vi "Fastlite5216_Example.vi"() -> ()   [LabVIEW 2020]
uses:
  <vilib>/Analysis/baseanly.llb/Mean (DBL).vi
  Fastlite5216_VIs/Fastlite5216-VIs.lvlib
  <vilib>/Analysis/NI_AALBase.lvlib
panel:
  in  "Correct Elec. Dark Current":bool
  in  "MeasConfigData":T1={"StartPixel"=0, "StopPixel"=2047, "Integration Time"=0.005, "Integration Delay"=0.0, "Trigger Mode"=enum."Software", "N StoreToRam"=0} {"Integration Delay" min=-0.02; "StopPixel" max=4095 step=1; "StartPixel" max=4095 step=1}
  out "Spectrum":cluster{dbl[], "Spectral DATA":dbl[]}[](graph)
  out "error out":errorcluster
  out "Black Pixels":u16[][](graph)
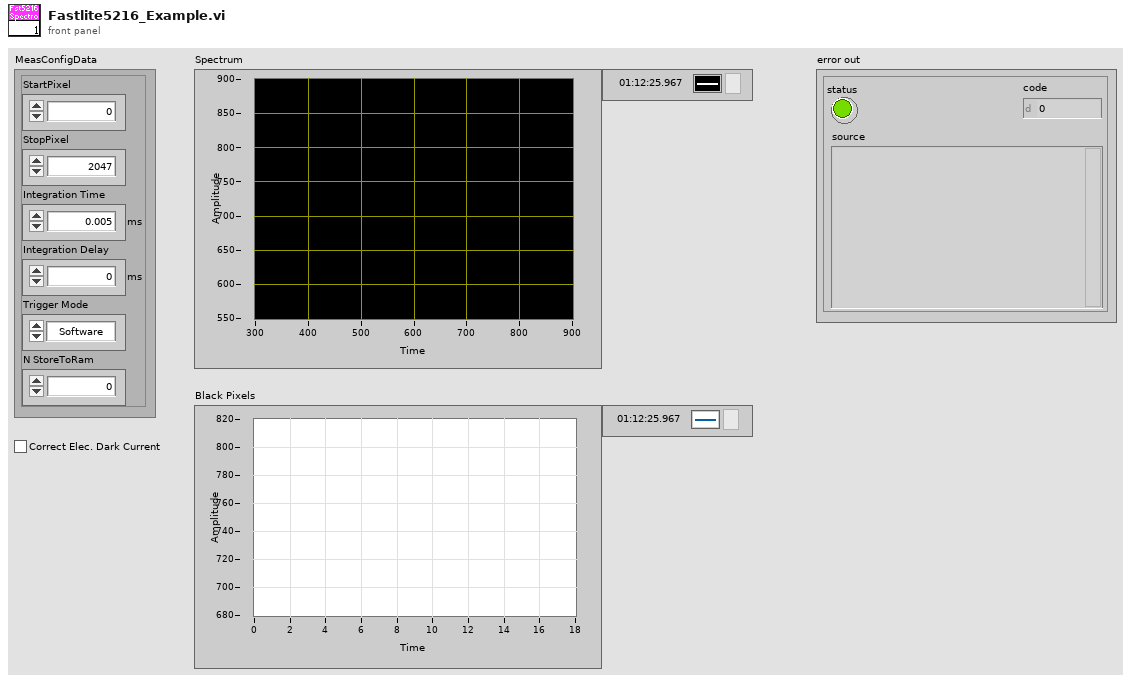
[diagram p1: front panel]
types:
  T1 = cluster{"StartPixel":u16, "StopPixel":u16, "Integration Time":sgl[unit], "Integration Delay":sgl[unit], "Trigger Mode":enum16{"Software", "Hardware"}, "N StoreToRam":u16}
  T2 = cluster{"VISA resource name":refnum<visa-resource-name>, "Serial ID":string, "FW Revision Nb":string}[]
  T3 = cluster{"VISA resource name":refnum<visa-resource-name>, "Serial ID":string, "FW Revision Nb":string}
  T4 = typedef "Fastlite5216-CTLs.lvlib/Fastlite5216_CTL_DeviceConfigData.ctl" = cluster{"Length":u16, "ConfigVersion":u16, "UserFriendly [64]":string, "Detector":T5, "Irradiance":T7, "Reflectance":T8, "SpectrumCorrection":T10, "Standalone":T11, "Temperature":cluster{"TempSensor 1":T18, "TempSensor 2":T18, "TempSensor 3":T18}, "TecControl":T19, "ProcessControl":T20, "Reserved":string}
  T5 = typedef "Fastlite5216-CTLs.lvlib/Fastlite5216_CTL_Detector.ctl" = cluster{"Sensor":T6, "NrPixels":u16, "Fit":cluster{"Order 0":sgl, "Order 1":sgl, "Order 2":sgl, "Order 3":sgl, "Order 4":sgl}, "NLEnable":u8, "NLCorrect":cluster{"NLCorrect 0":dbl, "NLCorrect 1":dbl, "NLCorrect 2":dbl, "NLCorrect 3":dbl, "NLCorrect 4":dbl, "NLCorrect 5":dbl, "NLCorrect 6":dbl, "NLCorrect 7":dbl}, "LowNLCounts":dbl, "HighNLCounts":dbl, "Gain":cluster{"Gain 0":sgl, "Gain 1":sgl}, "Reserved":sgl, "Offset":cluster{"Offset 0":sgl, "Offset 1":sgl}, "ExtOffset":sgl, "DefectivePixels":cluster{"DefectivePixels 0":u16, "DefectivePixels 1":u16, "DefectivePixels 2":u16, "DefectivePixels 3":u16, "DefectivePixels 4":u16, "DefectivePixels 5":u16, "DefectivePixels 6":u16, "DefectivePixels 7":u16, "DefectivePixels 8":u16, "DefectivePixels 9":u16, "DefectivePixels 10":u16, "DefectivePixels 11":u16, "DefectivePixels 12":u16, "DefectivePixels 13":u16, "DefectivePixels 14":u16, "DefectivePixels 15":u16, "DefectivePixels 16":u16, "DefectivePixels 17":u16, "DefectivePixels 18":u16, "DefectivePixels 19":u16, "DefectivePixels 20":u16, "DefectivePixels 21":u16, "DefectivePixels 22":u16, "DefectivePixels 23":u16, "DefectivePixels 24":u16, "DefectivePixels 25":u16, "DefectivePixels 26":u16, "DefectivePixels 27":u16, "DefectivePixels 28":u16, "DefectivePixels 29":u16}}
  T6 = typedef "Fastlite5216-CTLs.lvlib/Fastlite5216_CTL_Sensor.ctl" = enum8{"Reserved", "Hams8378-256", "Hams8378-1024", "ILX554", "Hams9201", "ToshibaTCD1304", "TSL1301", "TSL1401", "Hams8378-512", "Hams9840", "ILX511", "Hams10420-2048x64", "Hams11071-2048x64", "Hams7031-1024x122", "Hams7031-1024x58", "Hams11071-2048x16", "Hams11155", "SU256LSB", "SU512LDB", "Reserved2", "Reserved3", "HAMS11638", "HAMS11639", "HAMS12443", "HAMG9208_512", "HAMG13913", "HAMS13496"}
  T7 = typedef "Fastlite5216-CTLs.lvlib/Fastlite5216_CTL_Irradiance.ctl" = cluster{"IntensityCalib":T8, "CalibrationType":u8, "FiberDiameter":u32}
  T8 = typedef "Fastlite5216-CTLs.lvlib/Fastlite5216_CTL_SpectrumCalibration.ctl" = cluster{"Smoothing":T9, "CalIntTime":sgl, "CalibConvers":sgl[]}
  T9 = typedef "Fastlite5216-CTLs.lvlib/Fastlite5216_CTL_Smoothing.ctl" = cluster{"SmoothPix":u16, "SmoothModel":u8}
  T10 = typedef "Fastlite5216-CTLs.lvlib/Fastlite5216_CTL_SpectrumCorrection.ctl" = cluster{"SpectrumCorrect":sgl[]}
  T11 = typedef "Fastlite5216-CTLs.lvlib/Fastlite5216_CTL_Standalone.ctl" = cluster{"Enable":u8, "Meas":T12, "Nmsr":i16, "Standalone":T16}
  T12 = typedef "Fastlite5216-CTLs.lvlib/Fastlite5216_CTL_MeasConfigData.ctl" = cluster{"StartPixel":u16, "StopPixel":u16, "IntegrationTime":sgl, "IntegrationDelay":u32, "NrAverages":u32, "CorDynDark":T13, "Smoothing":T9, "SaturationDetection":u8, "Trigger":T14, "Control":T15}
  T13 = typedef "Fastlite5216-CTLs.lvlib/Fastlite5216_CTL_DarkCorrection.ctl" = cluster{"Enable":u8, "ForgetPercentage":u8}
  T14 = typedef "Fastlite5216-CTLs.lvlib/Fastlite5216_CTL_Trigger.ctl" = cluster{"Mode":u8, "Source":u8, "SourceType":u8}
  T15 = typedef "Fastlite5216-CTLs.lvlib/Fastlite5216_CTL_ControlSettings.ctl" = cluster{"StrobeControl":u16, "LaserDelay":u32, "LaserWidth":u32, "LaserWaveLength":sgl, "StoreToRam":u16}
  T16 = typedef "Fastlite5216-CTLs.lvlib/Fastlite5216_CTL_SDCard.ctl" = cluster{"Enable":u8, "SpectrumType":u8, "FileRootName [6]":cluster{"Char 1":u8, "Char 2":u8, "Char 3":u8, "Char 4":u8, "Char 5":u8, "Char 6":u8}, "TimeStamp":T17}
  T17 = typedef "Fastlite5216-CTLs.lvlib/Fastlite5216_CTL_TimeStamp.ctl" = cluster{"Time":u16, "Date":u16}
  T18 = typedef "Fastlite5216-CTLs.lvlib/Fastlite5216_CTL_TempSensor.ctl" = cluster{"Fit":cluster{"Order 0":sgl, "Order 1":sgl, "Order 2":sgl, "Order 3":sgl, "Order 4":sgl}}
  T19 = typedef "Fastlite5216-CTLs.lvlib/Fastlite5216_CTL_TecControl.ctl" = cluster{"Enable":u8, "SetPoint":sgl, "Fit":cluster{"Order 0":sgl, "Order 1":sgl}}
  T20 = typedef "Fastlite5216-CTLs.lvlib/Fastlite5216_CTL_ProcessControl.ctl" = cluster{"AnalogLow":cluster{"AnalogLow 1":sgl, "AnalogLow 2":sgl}, "AnalogHigh":cluster{"AnalogHigh 1":sgl, "AnalogHigh 2":sgl}, "DigitalLow":cluster{"DigitalLow 1":sgl, "DigitalLow 2":sgl, "DigitalLow 3":sgl, "DigitalLow 4":sgl, "DigitalLow 5":sgl, "DigitalLow 6":sgl, "DigitalLow 7":sgl, "DigitalLow 8":sgl, "DigitalLow 9":sgl, "DigitalLow 10":sgl}, "DigitalHigh":cluster{"DigitalHigh 1":sgl, "DigitalHigh 2":sgl, "DigitalHigh 3":sgl, "DigitalHigh 4":sgl, "DigitalHigh 5":sgl, "DigitalHigh 6":sgl, "DigitalHigh 7":sgl, "DigitalHigh 8":sgl, "DigitalHigh 9":sgl, "DigitalHigh 10":sgl}}
  T21 = cluster{"TimeStamp (s)":dbl, "Black Pixels":u16[], "Spectral DATA":u16[]}[]
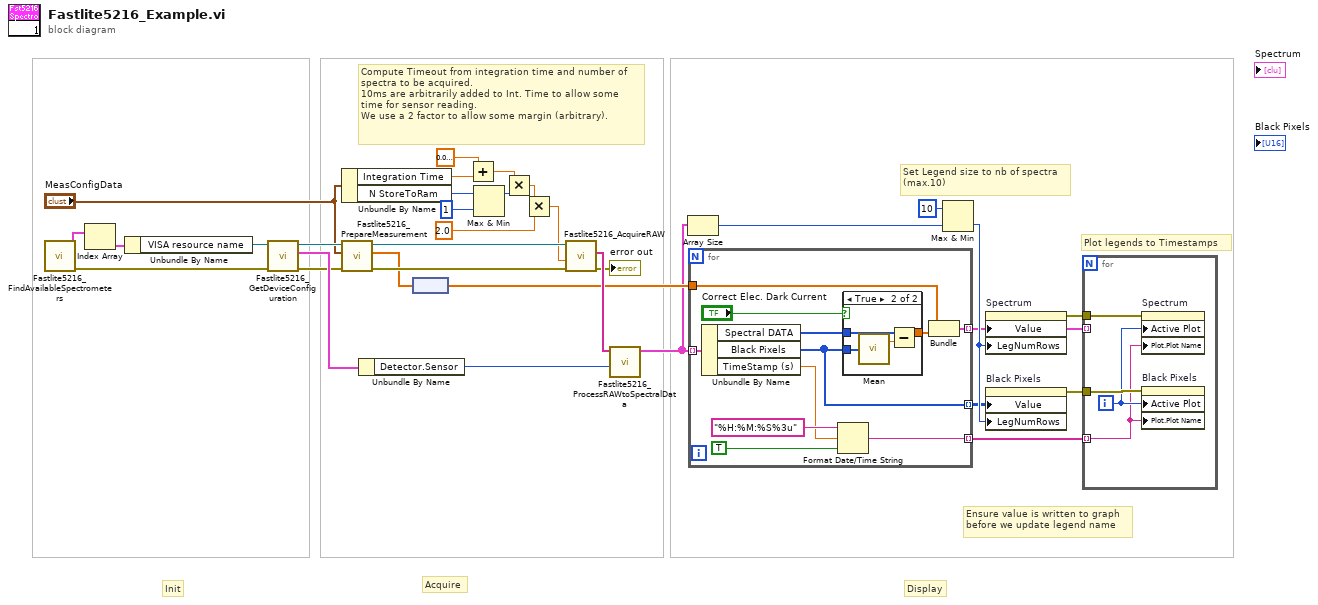
[diagram p0: block diagram]
diagram:
  # "Ensure value is written to graph\nbefore we update legend name"
  # "Acquire"
  # "Init"
  # "Display"
  # "Set Legend size to nb of spectra\n(max.10)"
  # "Plot legends to Timestamps"
  # "Compute Timeout from integration time and number of spectra to be acquired.\n10ms are arbitrarily added to Int. Time to allow some time for sensor reading.\nWe use a 2 factor to allow some margin (arbitrary)."
  n1 = call "Fastlite5216_FindAvailableSpectrometers.vi"() -> ("error out"=w26:errorcluster, "Spectro List"=w25:T2)  [unwired: 8 in, 2 out]
  n2 = Index Array(array=w25) -> (element=w24:T3)  [unwired: 1 in]
  n3 = Unbundle By Name(w24) -> ("VISA resource name"=w23:refnum<visa-resource-name>)
  n4 = call "Fastlite5216_GetDeviceConfiguration.vi"("error in (no error)"=w26, "Fastlite5216 VISA Resource In"=w23) -> ("error out"=w22:errorcluster, "DeviceConfigData"=w32:T4, "Fastlite5216 VISA Resource Out"=w33:refnum<visa-resource-name>)  [unwired: 6 in, 1 out]
  n5 = Unbundle By Name("MeasConfigData") -> ("Integration Time"=w16:sgl[unit], "N StoreToRam"=w15:u16)
  n6 = call "Fastlite5216_PrepareMeasurement.vi"("error in (no error)"=w22, "MeasConfigData"="MeasConfigData", "Fastlite5216 VISA Resource In"=w33) -> ("error out"=w30:errorcluster, "Wavelengths"=w18:dbl[unit][], "Fastlite5216 VISA Resource Out"=w31:refnum<visa-resource-name>)  [unwired: 6 in]
  n7 = Unbundle By Name(w32) -> ("Detector.Sensor"=w27:T6)
  n8 = node(w18) -> (w11:dbl[])
  n9 = Add(x=sgl[unit] 0.01, y=w16) -> (x+y=w8:sgl[unit])
  n10 = Max & Min(x=w15, y=u16 1) -> (max(x,y)=w2:u16)  [unwired: 1 out]
  n11 = Multiply(x=w8, y=w2) -> (x*y=w14:sgl[unit])
  n12 = Multiply(x=w14, y=sgl 2.0) -> (x*y=w12:sgl[unit])
  n13 = call "Fastlite5216_AcquireRAW.vi"("error in (no error)"=w30, "TimeOut"=w12, "Fastlite5216 VISA Resource In"=w31) -> ("error out"=→"error out":errorcluster, "Raw Spectral Data"=w29:string[])  [unwired: 4 in, 3 out]
  n14 = call "Fastlite5216_ProcessRAWtoSpectralData.vi"("Sensor"=w27, "Raw Spectral Data"=w29) -> ("Spectra"=w6:T21)  [unwired: 9 in]
  n15 = Array Size(array=w6) -> (size(s)=w5:i32)
  n16 = for {
    tunnel: w6 -> [w44] mode=indexing
    tunnel: [w36] -> w3 mode=indexing
    tunnel: [w38] -> w4 mode=indexing
    tunnel: [w42] -> w20 mode=indexing
    tunnel: w11 -> [w37]
    n17 = Unbundle By Name(w44) -> ("Spectral DATA"=w43:u16[], "Black Pixels"=w36:u16[], "TimeStamp (s)"=w39:dbl)
    n18 = Format Date/Time String(time format string (%c)="%H:%M:%S%3u", seconds (now)=w39, UTC format=TRUE) -> (date/time string=w42:string)
    n19 = case shown="True" "Correct Elec. Dark Current" {
      tunnel: w43 -> [w45 w49]
      tunnel: w36 -> [_ w48]
      tunnel: [w45 w47] -> w35
      frame False {
      }
      frame True {
        n20 = call-poly <vilib>:"Mean.vi"("X"=w48) -> ("mean"=w46:dbl)  [unwired: 1 out]
        n21 = Subtract(x=w49, y=w46) -> (x-y=w47:dbl[])
      }
    }
    n22 = Bundle(w37, "Spectral DATA"=w35) -> (w38:cluster{dbl[], "Spectral DATA":dbl[]})  [unwired: 1 in]
  }
  n23 = Max & Min(x=10 ("y"), y=w5) -> (min(x,y)=w9:i32)  [unwired: 1 out]
  n24 = property on="Spectrum" class="XYGraph (strict)"("Value"=w4, "LegNumRows"=w9) -> (error out=w21:errorcluster)  [unwired: 2 in, 1 out]
  n25 = property on="Black Pixels" class="WFGraph (strict)"("Value"=w3, "LegNumRows"=w9) -> (error out=w19:errorcluster)  [unwired: 2 in, 1 out]
  n26 = for {
    tunnel: w4 -> [_] mode=indexing
    tunnel: w20 -> [w50] mode=indexing
    tunnel: w21 -> [w53]
    tunnel: w19 -> [w52]
    i -> [w51]
    n27 = property on="Spectrum" class="XYGraph (strict)"(error in=w53, "Active Plot"=w51, "Plot.Plot Name"=w50) -> ()  [unwired: 1 in, 2 out]
    n28 = property on="Black Pixels" class="WFGraph (strict)"(error in=w52, "Active Plot"=w51, "Plot.Plot Name"=w50) -> ()  [unwired: 1 in, 2 out]
  }
